vi "Convert Keypress To Camera Movement.vi"(11 "ScanCode":i16) -> (2 "Camera Movement":T1, 3 "Move Camera":bool)   [LabVIEW 2020, in "Utility.lvlib"]
uses:
  Utility.lvlib
  Scene/Camera Movement.ctl
  Scene/Scene.lvclass
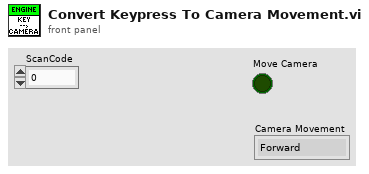
[diagram p1: front panel]
types:
  T1 = typedef "Scene.lvclass/Camera Movement.ctl" = enum16{"Forward", "Backwards", "Up", "Down", "Left", "Right", "Yaw CCW", "Yaw CW"}
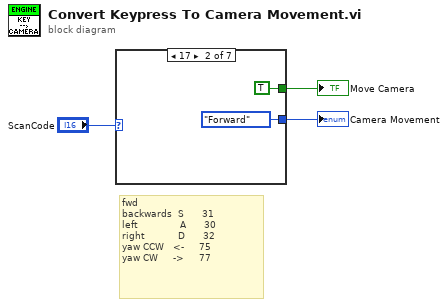
[diagram p0: block diagram]
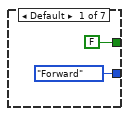
[diagram p2: hidden frame]
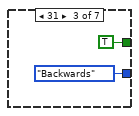
[diagram p3: hidden frame]
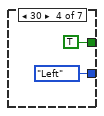
[diagram p4: hidden frame]
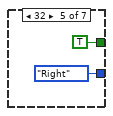
[diagram p5: hidden frame]
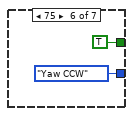
[diagram p6: hidden frame]
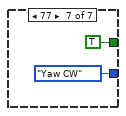
[diagram p7: hidden frame]
diagram:
  # "fwd    \nbackwards  S      31\nleft              A      30\nright           D      32\nyaw CCW   <-     75\nyaw CW     ->     77"
  n1 = case shown="17" "ScanCode" {
    tunnel: [Camera_Movement."Forward" ("Camera Movement") Camera_Movement."Forward" ("Camera Movement") Camera_Movement."Backwards" ("Camera Movement") Camera_Movement."Left" ("Camera Movement") Camera_Movement."Right" ("Camera Movement") Camera_Movement."Yaw CCW" ("Camera Movement") Camera_Movement."Yaw CW" ("Camera Movement")] -> w2
    tunnel: [FALSE TRUE TRUE TRUE TRUE TRUE TRUE] -> w1
    frame Default {
    }
    frame 17 {
    }
    frame 31 {
    }
    frame 30 {
    }
    frame 32 {
    }
    frame 75 {
    }
    frame 77 {
    }
  }
  "Camera Movement" <- w2
  "Move Camera" <- w1
